vi "Write MissionOp Index Msg.vi"(8 "error in (no error)":errorcluster, 10 "MissionOp Index":i32, 11 "Mission Set Op Index and Run Msg in":refnum<class "Mission Set Op Index and Run Msg.lvclass">) -> (0 "error out":errorcluster, 3 "Mission Set Op Index and Run Msg out":refnum<class "Mission Set Op Index and Run Msg.lvclass">)   [LabVIEW 2015, in "RDS Child Messages.lvlib" / "Mission Set Op Index and Run Msg.lvclass"]
uses:
  Mission Set Op Index and Run Msg.lvclass
  Mission Set Op Index and Run Msg.lvclass/Mission Set Op Index and Run Msg.ctl
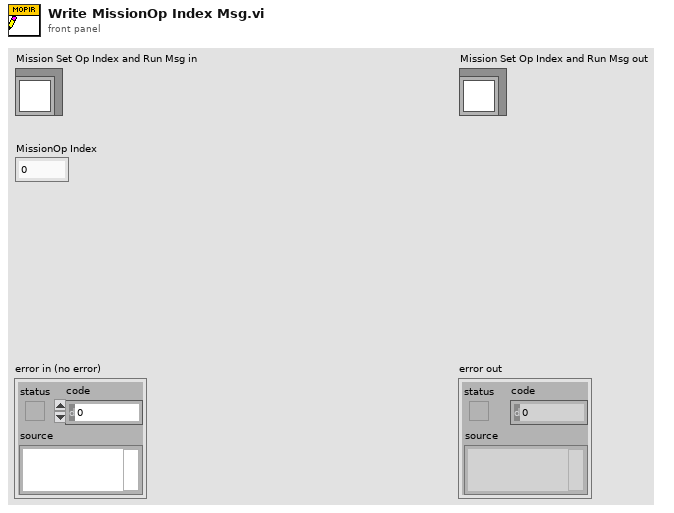
[diagram p1: front panel]
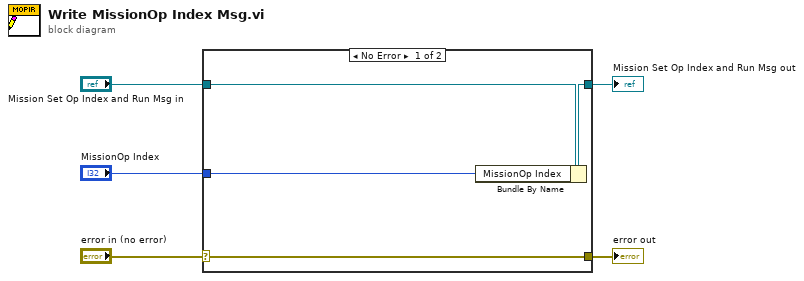
[diagram p0: block diagram]
diagram:
  n1 = case shown="No Error" "error in (no error)" {
    selector: "error in (no error)" -> [w9 w10]
    tunnel: [w9 w10] -> w4
    tunnel: [w7 w11] -> w2
    tunnel: "Mission Set Op Index and Run Msg in" -> [w8 w11]
    tunnel: "MissionOp Index" -> [w6 _]
    frame No Error {
      n2 = Bundle By Name(cluster=w8, "MissionOp Index"=w6) -> (w7:refnum<class "Mission Set Op Index and Run Msg.lvclass">)
    }
    frame Error {
    }
  }
  "error out" <- w4
  "Mission Set Op Index and Run Msg out" <- w2
